vi "Sensor Transformation.vi"(0 "Array":i32[](array[numeric])) -> ()   [LabVIEW 2018]
uses:
  <resource>/objmgr/IndComECAT.rc
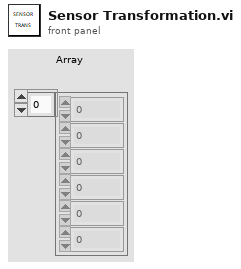
[diagram p1: front panel]
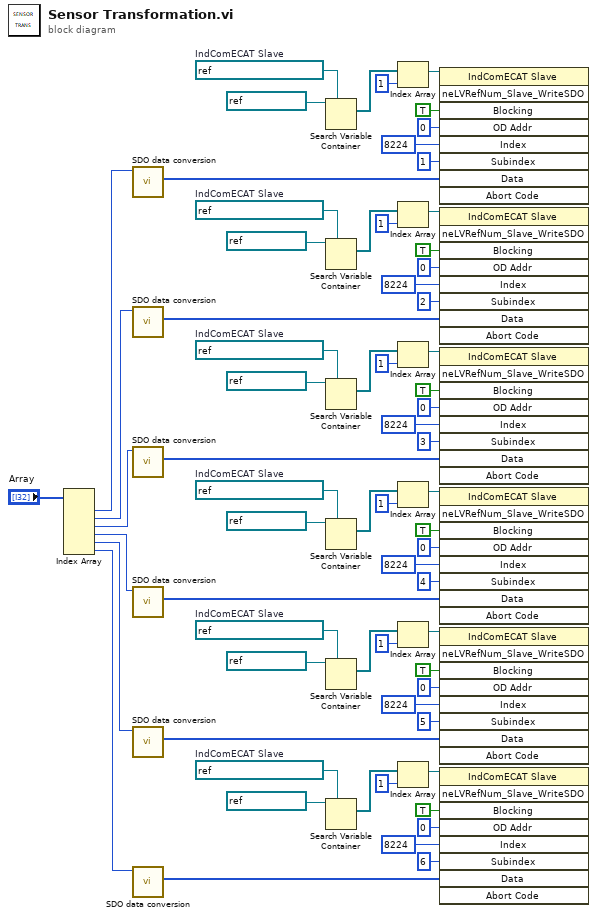
[diagram p0: block diagram]
diagram:
  w18 = refnum<k21> refnum  # IndComECAT Slave
  w21 = refnum<k21> refnum  # IndComECAT Slave
  w39 = refnum<k21> refnum  # IndComECAT Slave
  w36 = refnum<k21> refnum  # IndComECAT Slave
  w54 = refnum<k21> refnum  # IndComECAT Slave
  w60 = refnum<k21> refnum  # IndComECAT Slave
  n1 = Index Array(array="Array") -> (element #1=w56:i32, element #2=w5:i32, element #3=w4:i32, element #4=w3:i32, element #5=w2:i32, element #6=w1:i32)  [unwired: 6 in]
  n2 = call "SDO data conversion.vi"("Decimal Input"=w56) -> ("Array"=w58:u8[])  [unwired: 9 in, 1 out]
  n3 = call "SDO data conversion.vi"("Decimal Input"=w5) -> ("Array"=w7:u8[])  [unwired: 9 in, 1 out]
  n4 = call "SDO data conversion.vi"("Decimal Input"=w4) -> ("Array"=w8:u8[])  [unwired: 9 in, 1 out]
  n5 = call "SDO data conversion.vi"("Decimal Input"=w3) -> ("Array"=w6:u8[])  [unwired: 9 in, 1 out]
  n6 = call "SDO data conversion.vi"("Decimal Input"=w2) -> ("Array"=w9:u8[])  [unwired: 9 in, 1 out]
  n7 = call "SDO data conversion.vi"("Decimal Input"=w1) -> ("Array"=w10:u8[])  [unwired: 9 in, 1 out]
  n8 = Search Variable Container(7:w60, 11:refnum<k21> "ni.var.io:/" ("container refnum in")) -> (2:w62:refnum<k21>[])  [unwired: 4 in, 2 out]
  n9 = Search Variable Container(7:w54, 11:refnum<k21> "ni.var.io:/" ("container refnum in")) -> (2:w52:refnum<k21>[])  [unwired: 4 in, 2 out]
  n10 = Search Variable Container(7:w36, 11:refnum<k21> "ni.var.io:/" ("container refnum in")) -> (2:w34:refnum<k21>[])  [unwired: 4 in, 2 out]
  n11 = Search Variable Container(7:w39, 11:refnum<k21> "ni.var.io:/" ("container refnum in")) -> (2:w41:refnum<k21>[])  [unwired: 4 in, 2 out]
  n12 = Search Variable Container(7:w21, 11:refnum<k21> "ni.var.io:/" ("container refnum in")) -> (2:w23:refnum<k21>[])  [unwired: 4 in, 2 out]
  n13 = Search Variable Container(7:w18, 11:refnum<k21> "ni.var.io:/" ("container refnum in")) -> (2:w16:refnum<k21>[])  [unwired: 4 in, 2 out]
  n14 = Index Array(array=w62, index=1) -> (element=w61:refnum<k21>)
  n15 = Index Array(array=w52, index=1) -> (element=w53:refnum<k21>)
  n16 = Index Array(array=w34, index=1) -> (element=w35:refnum<k21>)
  n17 = Index Array(array=w41, index=1) -> (element=w40:refnum<k21>)
  n18 = Index Array(array=w23, index=1) -> (element=w22:refnum<k21>)
  n19 = Index Array(array=w16, index=1) -> (element=w17:refnum<k21>)
  n20 = invoke class="IndComECAT Slave" method="neLVRefNum_Slave_WriteSDO"(reference=w61, "Blocking"=TRUE, "OD Addr"=u16 0, "Index"=u16 8224, "Subindex"=u8 1, "Data"=w58) -> ()  [unwired: 3 in, 9 out]
  n21 = invoke class="IndComECAT Slave" method="neLVRefNum_Slave_WriteSDO"(reference=w53, "Blocking"=TRUE, "OD Addr"=u16 0, "Index"=u16 8224, "Subindex"=u8 2, "Data"=w7) -> ()  [unwired: 3 in, 9 out]
  n22 = invoke class="IndComECAT Slave" method="neLVRefNum_Slave_WriteSDO"(reference=w35, "Blocking"=TRUE, "OD Addr"=u16 0, "Index"=u16 8224, "Subindex"=u8 3, "Data"=w8) -> ()  [unwired: 3 in, 9 out]
  n23 = invoke class="IndComECAT Slave" method="neLVRefNum_Slave_WriteSDO"(reference=w40, "Blocking"=TRUE, "OD Addr"=u16 0, "Index"=u16 8224, "Subindex"=u8 4, "Data"=w6) -> ()  [unwired: 3 in, 9 out]
  n24 = invoke class="IndComECAT Slave" method="neLVRefNum_Slave_WriteSDO"(reference=w22, "Blocking"=TRUE, "OD Addr"=u16 0, "Index"=u16 8224, "Subindex"=u8 5, "Data"=w9) -> ()  [unwired: 3 in, 9 out]
  n25 = invoke class="IndComECAT Slave" method="neLVRefNum_Slave_WriteSDO"(reference=w17, "Blocking"=TRUE, "OD Addr"=u16 0, "Index"=u16 8224, "Subindex"=u8 6, "Data"=w10) -> ()  [unwired: 3 in, 9 out]
